vi "Create Variant Dictionary from Variant Cluster.vi"(8 "error in (no error)":errorcluster, 11 "Variant in":variant) -> (0 "error out":errorcluster, 3 "Variant out":variant)   [LabVIEW 2018, in "ClientMessaging.lvlib"]
uses:
  ClientMessaging.lvlib
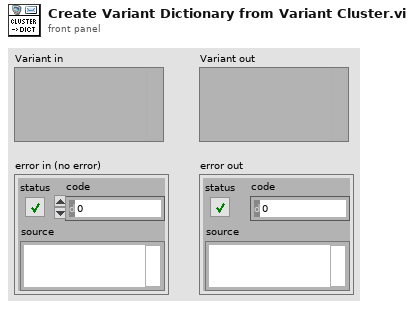
[diagram p1: front panel]
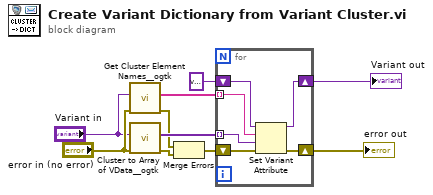
[diagram p0: block diagram]
diagram:
  n1 = call <userlib>:"Get Cluster Element Names__ogtk.vi"("error in (no error)"="error in (no error)", "Cluster"="Variant in") -> ("error out"=w4:errorcluster, "Element Names"=w6:string[])  [unwired: 8 in]
  n2 = call <userlib>:"Cluster to Array of VData__ogtk.vi"("error in (no error)"="error in (no error)", "Cluster"="Variant in") -> ("error out"=w3:errorcluster, "Array of VData"=w5:variant[])  [unwired: 8 in]
  n3 = Merge Errors(w4, w3) -> (w2:errorcluster)
  n4 = for {
    tunnel: w6 -> [w15] mode=indexing
    tunnel: w5 -> [w11] mode=indexing
    shift-right: [w13] -> w9
    shift-left: w2 -> [w12]
    shift-right: [w14] -> w10
    shift-left: variant -> [w16]
    n5 = Set Variant Attribute(Variant=w16, name=w15, value=w11, error in=w12) -> (Variant out=w14:variant, error out=w13:errorcluster)  [unwired: 1 out]
  }
  "Variant out" <- w10
  "error out" <- w9
